vi "cross_product.vi"(1 "b":cluster{dbl, dbl, dbl}, 2 "a":cluster{dbl, dbl, dbl}) -> (0 "a cross b":cluster{dbl, dbl, dbl})   [LabVIEW 2015]
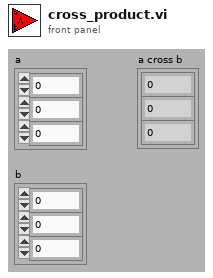
[diagram p1: front panel]
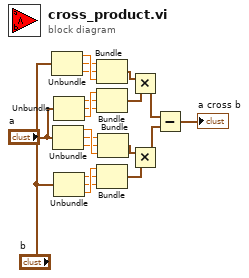
[diagram p0: block diagram]
diagram:
  n1 = Unbundle("b") -> (w12:dbl, w10:dbl, w11:dbl)
  n2 = Unbundle("a") -> (w3:dbl, w1:dbl, w2:dbl)
  n3 = Unbundle("a") -> (w8:dbl, w7:dbl, w9:dbl)
  n4 = Unbundle("b") -> (w5:dbl, w4:dbl, w6:dbl)
  n5 = Bundle(w10, w11, w12) -> (w14:cluster{dbl, dbl, dbl})  [unwired: 1 out]
  n6 = Bundle(w9, w8, w7) -> (w13:cluster{dbl, dbl, dbl})  [unwired: 1 out]
  n7 = Bundle(w6, w5, w4) -> (w16:cluster{dbl, dbl, dbl})  [unwired: 1 out]
  n8 = Bundle(w1, w2, w3) -> (w15:cluster{dbl, dbl, dbl})  [unwired: 1 out]
  n9 = Multiply(x=w14, y=w13) -> (x*y=w17:cluster{dbl, dbl, dbl})
  n10 = Multiply(x=w15, y=w16) -> (x*y=w18:cluster{dbl, dbl, dbl})
  n11 = Subtract(x=w17, y=w18) -> (x-y=→"a cross b":cluster{dbl, dbl, dbl})
